vi "Run.vi"(8 "error in (no error)":errorcluster, 11 "Assembler in":refnum<class "Assembler.lvclass">) -> (0 "error out":errorcluster, 3 "Assembler out":refnum<class "Assembler.lvclass">)   [LabVIEW 2016, in "CLD Exam - Car Wash.lvlib" / "Assembler.lvclass"]
uses:
  Assembler.lvclass
  Assembler.lvclass/Assembler.ctl
  Car Position Simulator/Car Position Simulator.lvclass
  Car Wash Console/Car Wash Console.lvclass
  Car Wash Display/Car Wash Display.lvclass
  Car Wash Station Sequencer/Car Wash Station Sequencer.lvclass
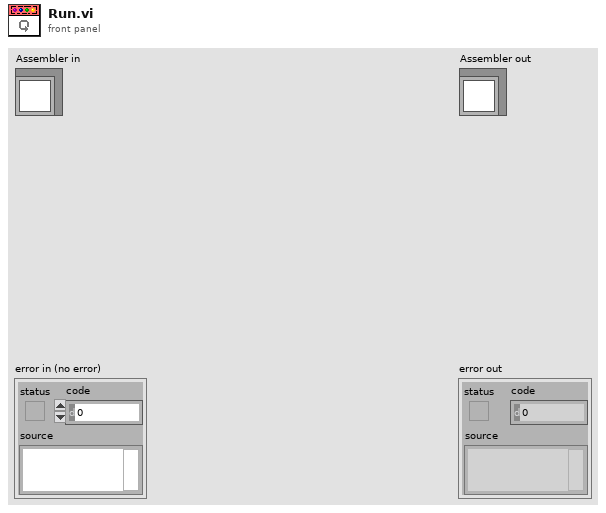
[diagram p1: front panel]
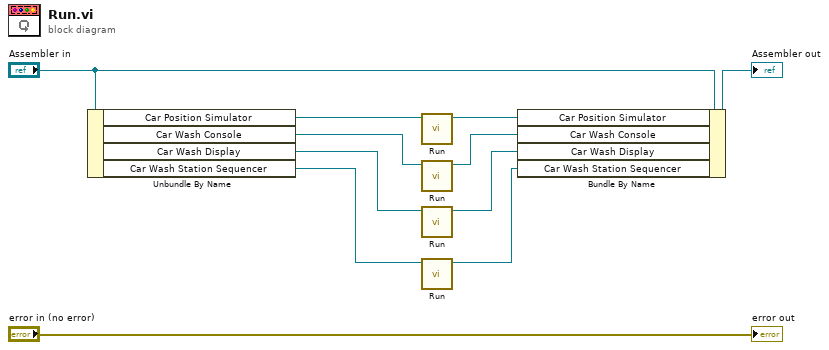
[diagram p0: block diagram]
diagram:
  n1 = Unbundle By Name("Assembler in") -> ("Car Position Simulator"=w10:refnum<class "Car Position Simulator.lvclass">, "Car Wash Console"=w6:refnum<class "Car Wash Console.lvclass">, "Car Wash Display"=w4:refnum<class "Car Wash Display.lvclass">, "Car Wash Station Sequencer"=w2:refnum<class "Car Wash Station Sequencer.lvclass">)
  n2 = call-dynamic "Run.vi"("Car Position Simulator in"=w10) -> ("Car Position Simulator out"=w7:refnum<class "Car Position Simulator.lvclass">)  [unwired: 9 in, 1 out]
  n3 = call-dynamic "Run.vi"("Car Wash Console in"=w6) -> ("Car Wash Console out"=w5:refnum<class "Car Wash Console.lvclass">)  [unwired: 9 in, 1 out]
  n4 = call-dynamic "Run.vi"("Car Wash Console in"=w4) -> ("Car Wash Console out"=w3:refnum<class "Car Wash Display.lvclass">)  [unwired: 9 in, 1 out]
  n5 = call-dynamic "Run.vi"("Car Wash Station Sequencer in"=w2) -> ("Car Wash Station Sequencer out"=w1:refnum<class "Car Wash Station Sequencer.lvclass">)  [unwired: 9 in, 1 out]
  n6 = Bundle By Name(cluster="Assembler in", "Car Position Simulator"=w7, "Car Wash Console"=w5, "Car Wash Display"=w3, "Car Wash Station Sequencer"=w1) -> (→"Assembler out":refnum<class "Assembler.lvclass">)
  "error out" <- "error in (no error)"
